vi "Estimated Time Required.vi"(1 "Lithography Data":T1(array[cluster])) -> (0 "Estimated Time Required":timestamp format="%<%I:%M:%S>T")   [LabVIEW 2013]
doc: "Calculates the time required to complete lithography."
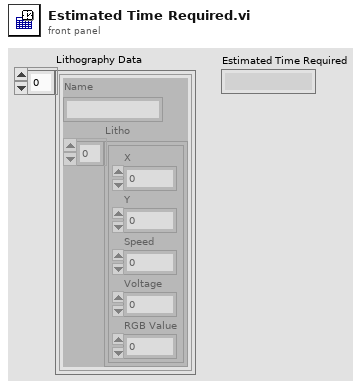
[diagram p1: front panel]
types:
  T1 = cluster{"Name":string, "Litho":cluster{"X":dbl, "Y":dbl, "Speed":dbl, "Voltage":dbl, "RGB Value":dbl}[]}[]
  T2 = cluster{"X":dbl, "Y":dbl, "Speed":dbl, "Voltage":dbl, "RGB Value":dbl}[]
  T3 = cluster{"X":dbl, "Y":dbl, "Speed":dbl, "Voltage":dbl, "RGB Value":dbl}
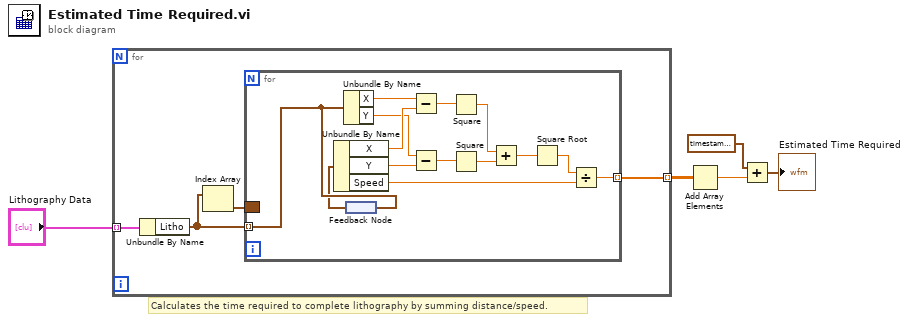
[diagram p0: block diagram]
diagram:
  # "Calculates the time required to complete lithography by summing distance/speed."
  n1 = for {
    tunnel: "Lithography Data" -> [w9] mode=indexing
    tunnel: [w6] -> w2 mode=indexing
    n2 = Unbundle By Name(w9) -> ("Litho"=w8:T2)
    n3 = Index Array(array=w8) -> (element=w7:T3)  [unwired: 1 in]
    n4 = for {
      tunnel: w8 -> [w18] mode=indexing
      border: w7 -> [_]
      tunnel: [w19] -> w6 mode=indexing
      n5 = Unbundle By Name(w18) -> ("X"=w16:dbl, "Y"=w13:dbl)
      n6 = feedback-in #1(w18) -> ()
      n7 = feedback #1() -> (w17:T3)
      n8 = Unbundle By Name(w17) -> ("X"=w15:dbl, "Y"=w12:dbl, "Speed"=w10:dbl)
      n9 = Subtract(x=w16, y=w15) -> (x-y=w14:dbl)
      n10 = Subtract(x=w13, y=w12) -> (x-y=w11:dbl)
      n11 = Square(x=w14) -> (x^2=w23:dbl)
      n12 = Square(x=w11) -> (x^2=w22:dbl)
      n13 = Add(x=w23, y=w22) -> (x+y=w21:dbl)
      n14 = Square Root(x=w21) -> (sqrt(x)=w20:dbl)
      n15 = Divide(x=w20, y=w10) -> (x/y=w19:dbl)
    }
  }
  n16 = Add Array Elements(numeric array=w2) -> (sum=w4:dbl)
  n17 = Add(x=timestamp(-68400 s since 1904-01-01), y=w4) -> (x+y=→"Estimated Time Required":timestamp)
